vi "Teleop.vi"(10 "Match Info":T1={"Autonomous Elapsed Seconds"=0.0, "TeleOp Elapsed Seconds"=100.423, "Disabled Elapsed Seconds"=64.63, "Visited Autonomous"=FALSE, "Visited TeleOp"=TRUE, "Visited Disabled"=TRUE, "Autonomous Settings"={"Autonomous Style"=enum."Independent", "VI Refnum"=refnum}}, 11 "Call Context":T2=enum."Stop") -> ()   [LabVIEW 2015]
doc: "This VI is called for each TeleOp packet received from the DS where the robot is not disabled. It is often used to read from the joysticks and update I/O or to update setpoints for timed control loops. It should complete and return within 20 milliseconds or it may miss DS packets."
uses:
  <vilib>/Rock Robotics/WPI/DriverStation/WPI_DriverStationDerivedRobotMode.ctl
  <vilib>/Rock Robotics/WPI/DriverStation/WPI_DriverStationMatch Info.ctl
  <vilib>/Rock Robotics/WPI/Utilities/WPI_GetSetVariantRefNum.vi
  <vilib>/addons/control/pid/pid.llb/PID Output Rate Limiter (DBL).vi
  <vilib>/addons/control/pid/NI_PID_pid.lvlib
panel:
  in  "Far":dbl=0.7
  in  "Close":dbl=0.7
  in  "Target":dbl
  in  "P":dbl=1.0 format="%#_13g"
  in  "I":dbl format="%#_13g"
  in  "dT":dbl format="%#_13g"
  out "Right Chart":dbl(graph)
  out "Left Chart":dbl(graph)
  in  "dt (s)":dbl=2.0 format="%.2f"
  in  "output rate (EGU/min)":dbl=25.0 format="%.2f"
  in  "initial output":dbl format="%.2f"
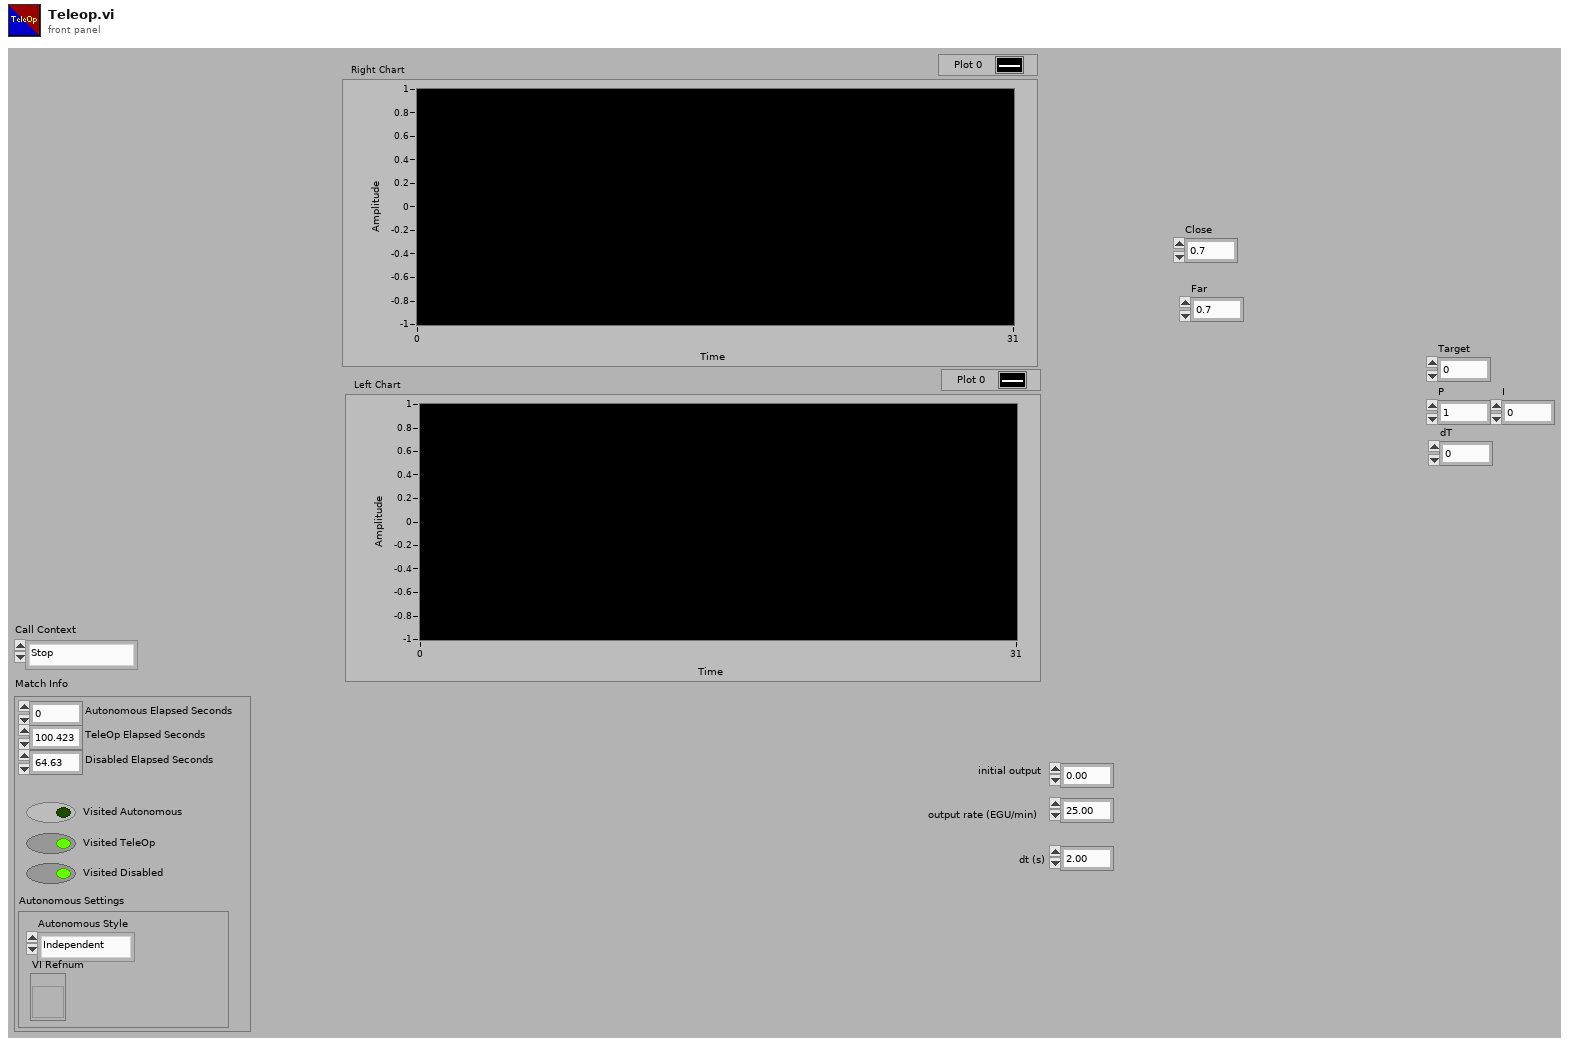
[diagram p1: front panel]
types:
  T1 = typedef "WPI_DriverStationMatch Info.ctl" = cluster{"Autonomous Elapsed Seconds":dbl, "TeleOp Elapsed Seconds":dbl, "Disabled Elapsed Seconds":dbl, "Visited Autonomous":bool, "Visited TeleOp":bool, "Visited Disabled":bool, "Autonomous Settings":cluster{"Autonomous Style":enum16{"Iterative", "Independent"}, "VI Refnum":refnum<vi>}}
  T2 = typedef "WPI_DriverStationDerivedRobotMode.ctl" = enum16{"Init", "Execute", "Stop"}
  T3 = typedef "WPI_JoystickDevRef.ctl" = cluster{"Device":T4}
  T4 = typedef "WPI_JoystickDeviceEnum.ctl" = enum16{"USB 0", "USB 1", "USB 2", "USB 3", "USB 4", "USB 5"}
  T5 = typedef "WPI_RobotDriveDevRef.ctl" = cluster{"DevStatus":errorcluster, "Motors[]":T6[], "Square Inputs":bool, "Max Output":dbl}
  T6 = typedef "WPI_MotorControlDeviceRef.ctl" = cluster{"DeviceStatus":errorcluster, "Type":T7, "PWM":cluster{"PWM Channel":T8, "DeadBand":T9}, "CAN":cluster{"Device Number":u8, "Control Mode":T10, "Semaphore":T11, "Max Vout":dbl, "TalonSRX Control Mode":T12}, "Invert":bool}
  T7 = typedef "WPI_MotorControlType.ctl" = enum16{"PWM", "CAN", "CANTalonSRX"}
  T8 = typedef "FPGA_DIOPWMChannel.ctl" = enum8{"PWM 0", "PWM 1", "PWM 2", "PWM 3", "PWM 4", "PWM 5", "PWM 6", "PWM 7", "PWM 8", "PWM 9", "PWM MXP 0", "PWM MXP 1", "PWM MXP 2", "PWM MXP 3", "PWM MXP 4", "PWM MXP 5", "PWM MXP 6", "PWM MXP 7", "PWM MXP 8", "PWM MXP 9", "Invalid"}
  T9 = typedef "WPI_PWMDeadband.ctl" = cluster{"Name":string, "maxPositivePwm":i32, "minPositivePwm":i32, "centerPwm":i32, "maxNegativePwm":i32, "minNegativePwm":i32, "angularRange":u16}
  T10 = typedef "WPI_CANJaguar_ControlMode.ctl" = enum8{"Percent VBus", "Current", "Speed", "Position", "Voltage"}
  T11 = typedef "Semaphore RefNum" = refnum<k1>
  T12 = typedef "WPI_CANTalonSRX_APIControlMode.ctl" = enum8{"Percent VBus", "Speed", "Position", "Slave", "Unchanged / Invalid", "Voltage Compensation", "Current", "Motion Profile"}
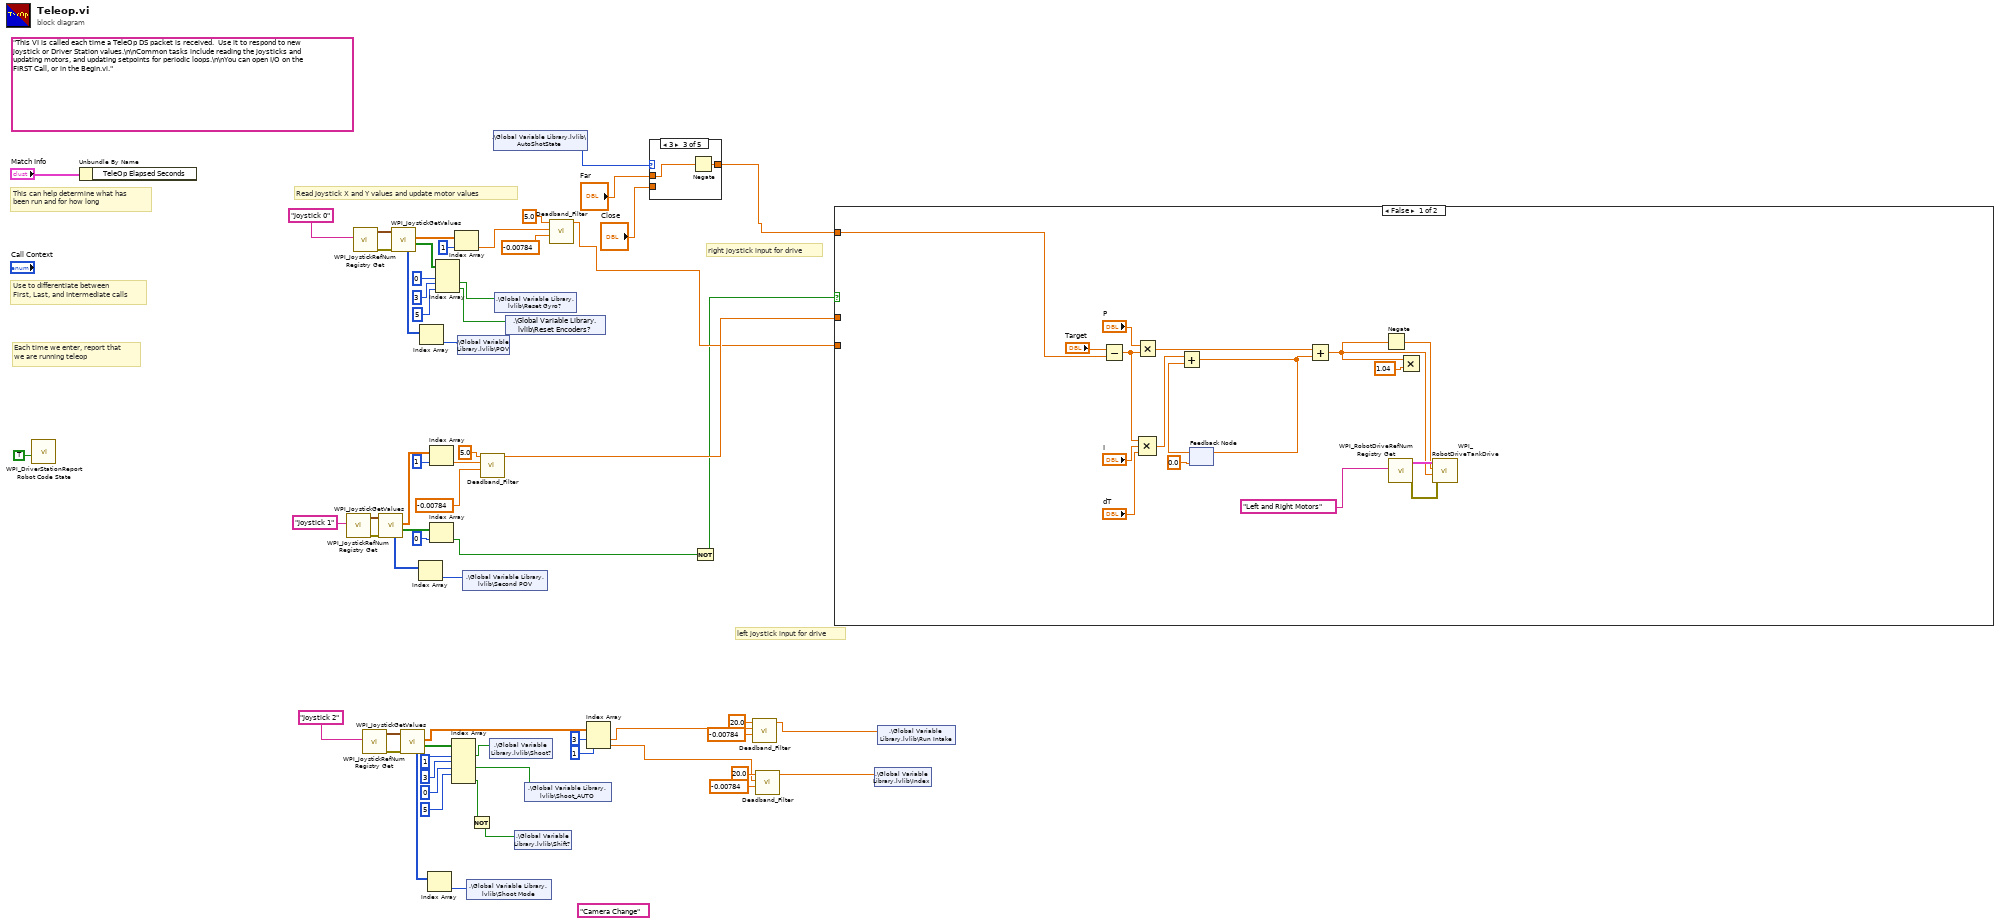
[diagram p0: block diagram]
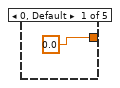
[diagram p2: hidden frame]
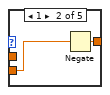
[diagram p3: hidden frame]
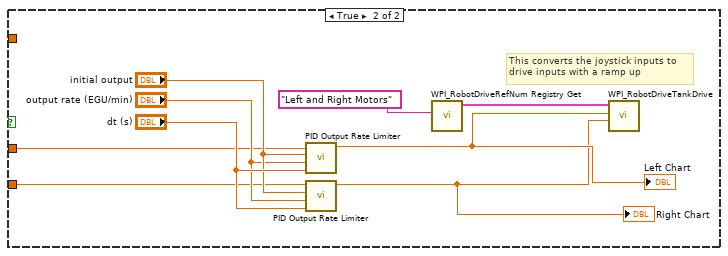
[diagram p6: hidden frame]
diagram:
  (unwired) "Camera Change" ("Name")
  (unwired) "This VI is called each time a TeleOp DS packet is received.  Use it to respond to new joystick or Driver Station values.\n\nCommon tasks include reading the joysticks and updating motors, and updating setpoints for periodic loops.\n\nYou can open I/O on the FIRST Call, or in the Begin.vi."
  # "left joystick input for drive"
  # "right joystick input for drive"
  # "Each time we enter, report that\nwe are running teleop"
  # "Use to differentiate between\nFirst, Last, and Intermediate calls"
  # "This can help determine what has\nbeen run and for how long"
  # "Read Joystick X and Y values and update motor values"
  n1 = call <vilib>:"WPI_DriverStationReport Robot Code State.vi"("TeleOp"=TRUE ("Autonomous")) -> ()  [unwired: 10 in, 1 out]
  n2 = Unbundle By Name("Match Info") -> ()  [unwired: 1 out]
  n3 = call <vilib>:"WPI_JoystickRefNum Registry Get.vi"("refnum name"="Joystick 1") -> ("error out"=w52:errorcluster, "JoystickDevRef"=w51:T3)  [unwired: 1 in, 8 out]
  n4 = call <vilib>:"WPI_JoystickRefNum Registry Get.vi"("refnum name"="Joystick 0") -> ("error out"=w58:errorcluster, "JoystickDevRef"=w57:T3)  [unwired: 1 in, 8 out]
  n5 = call <vilib>:"WPI_JoystickRefNum Registry Get.vi"("refnum name"="Joystick 2") -> ("error out"=w49:errorcluster, "JoystickDevRef"=w48:T3)  [unwired: 1 in, 8 out]
  n6 = call <vilib>:"WPI_JoystickGetValues.vi"("error in (no error)"=w52, "JoystickDevRef"=w51) -> ("Buttons"=w8:bool[], "Axes"=w50:dbl[], "POVs"=w31:i16[])  [unwired: 5 in, 2 out]
  n7 = call <vilib>:"WPI_JoystickGetValues.vi"("error in (no error)"=w58, "JoystickDevRef"=w57) -> ("Buttons"=w55:bool[], "Axes"=w56:dbl[], "POVs"=w54:i16[])  [unwired: 5 in, 2 out]
  n8 = call <vilib>:"WPI_JoystickGetValues.vi"("error in (no error)"=w49, "JoystickDevRef"=w48) -> ("Buttons"=w47:bool[], "Axes"=w27:dbl[], "POVs"=w34:i16[])  [unwired: 5 in, 2 out]
  n9 = Index Array(array=w31) -> (element=w30:i16)  [unwired: 1 in]
  n10 = Index Array(array=w54) -> (element=w53:i16)  [unwired: 1 in]
  n11 = Index Array(array=w34) -> (element=w33:i16)  [unwired: 1 in]
  n12 = Index Array(array=w50, index=1) -> (element=w40:dbl)
  n13 = Index Array(array=w8, index=0) -> (element=w6:bool)
  n14 = Index Array(array=w55, index #1=0 ("index"), index #2=3 ("index"), index #3=5 ("index")) -> (element #2=w32:bool, element #3=w14:bool)  [unwired: 1 out]
  n15 = Index Array(array=w47, index #1=1 ("index"), index #2=3 ("index"), index #3=0 ("index"), index #4=5 ("index")) -> (element #1=w46:bool, element #3=w11:bool, element #5=w10:bool)  [unwired: 1 in, 2 out]
  n16 = Index Array(array=w56, index=1) -> (element=w35:dbl)
  n17 = shared-variable ".\\Global Variable Library.lvlib\\POV"(w53) -> ()  [unwired: 1 in, 1 out]
  n18 = shared-variable ".\\Global Variable Library.lvlib\\Second POV"(w30) -> ()  [unwired: 1 in, 1 out]
  n19 = shared-variable ".\\Global Variable Library.lvlib\\Shoot Mode"(w33) -> ()  [unwired: 1 in, 1 out]
  n20 = Not(x=w10) -> (.not. x?=w9:bool)
  n21 = call "Deadband_Filter.vi"("Deadband_Center"=-0.00784, "Input"=w40, "Deadband_Size(%)"=5.0) -> ("Deadbanded_Output"=w13:dbl)  [unwired: 8 in]
  n22 = shared-variable ".\\Global Variable Library.lvlib\\Shoot?"(w46) -> ()  [unwired: 1 in, 1 out]
  n23 = shared-variable ".\\Global Variable Library.lvlib\\AutoShotState"() -> (w3:u32)  [unwired: 1 in, 1 out]
  n24 = shared-variable ".\\Global Variable Library.lvlib\\Reset Gyro?"(w32) -> ()  [unwired: 1 in, 1 out]
  n25 = shared-variable ".\\Global Variable Library.lvlib\\Reset Encoders?"(w14) -> ()  [unwired: 1 in, 1 out]
  n26 = shared-variable ".\\Global Variable Library.lvlib\\Shift?"(w9) -> ()  [unwired: 1 in, 1 out]
  n27 = shared-variable ".\\Global Variable Library.lvlib\\Shoot_AUTO"(w11) -> ()  [unwired: 1 in, 1 out]
  n28 = call "Deadband_Filter.vi"("Deadband_Center"=-0.00784, "Input"=w35, "Deadband_Size(%)"=5.0) -> ("Deadbanded_Output"=w12:dbl)  [unwired: 8 in]
  n29 = Index Array(array=w27, index #1=3 ("index"), index #2=1 ("index")) -> (element #1=w20:dbl, element #2=w17:dbl)
  n30 = case shown="3" w3 {
    tunnel: [0.0 w66 w68 w69 w70] -> w4
    tunnel: "Far" -> [_ _ w67 _ w70]
    tunnel: "Close" -> [_ w65 _ w69 _]
    frame 0, Default {
    }
    frame 1 {
      n31 = Negate(x=w65) -> (-x=w66:dbl)
    }
    frame 3 {
      n32 = Negate(x=w67) -> (-x=w68:dbl)
    }
    frame 4 {
    }
    frame 6 {
    }
  }
  n33 = Not(x=w6) -> (.not. x?=w5:bool)
  n34 = call "Deadband_Filter.vi"("Deadband_Center"=-0.00784, "Input"=w20, "Deadband_Size(%)"=20.0) -> ("Deadbanded_Output"=w21:dbl)  [unwired: 8 in]
  n35 = call "Deadband_Filter.vi"("Deadband_Center"=-0.00784, "Input"=w17, "Deadband_Size(%)"=20.0) -> ("Deadbanded_Output"=w16:dbl)  [unwired: 8 in]
  n36 = case shown="False" w5 {
    tunnel: w13 -> [_ w91]
    tunnel: w12 -> [_ w90]
    tunnel: w4 -> [w73 _]
    frame False {
      n37 = Subtract(x="Target", y=w73) -> (x-y=w81:dbl)
      n38 = Multiply(x="P", y=w81) -> (x*y=w84:dbl)
      n39 = Compound Arithmetic op=MULTIPLY(w81, "I", "dT") -> (w76:dbl)
      n40 = feedback #1(0.0) -> (w77:dbl)
      n41 = Add(x=w76, y=w77) -> (x+y=w78:dbl)
      n42 = feedback-in #1(w78) -> ()
      n43 = Add(x=w84, y=w78) -> (x+y=w72:dbl)
      n44 = Negate(x=w72) -> (-x=w71:dbl)
      n45 = call <vilib>:"WPI_RobotDriveRefNum Registry Get.vi"("refnum name"="Left and Right Motors") -> ("error out"=w86:errorcluster, "RobotDriveDevRef"=w85:T5)  [unwired: 9 in]
      n46 = Multiply(x=w72, y=1.04) -> ()  [unwired: 1 out]
      n47 = call <vilib>:"WPI_RobotDriveTankDrive.vi"("error in (no error)"=w86, "Right axis value"=w72, "Left axis value"=w71, "RobotDriveDevRef"=w85) -> ()  [unwired: 5 in, 3 out]
    }
    frame True {
      # "This converts the joystick inputs to\ndrive inputs with a ramp up"
      n48 = call-poly <vilib>:"PID Output Rate Limiter.vi"("dt (s)"="dt (s)", "output rate (EGU/min)"="output rate (EGU/min)", "initial output"="initial output", "input (controller output)"=w91) -> ("output"=w89:dbl)  [unwired: 4 in, 1 out]
      "Left Chart" <- w89
      n49 = call-poly <vilib>:"PID Output Rate Limiter.vi"("dt (s)"="dt (s)", "output rate (EGU/min)"="output rate (EGU/min)", "initial output"="initial output", "input (controller output)"=w90) -> ("output"=w88:dbl)  [unwired: 4 in, 1 out]
      "Right Chart" <- w88
      n50 = call <vilib>:"WPI_RobotDriveRefNum Registry Get.vi"("refnum name"="Left and Right Motors") -> ("RobotDriveDevRef"=w95:T5)  [unwired: 9 in, 1 out]
      n51 = call <vilib>:"WPI_RobotDriveTankDrive.vi"("Right axis value"=w88, "Left axis value"=w89, "RobotDriveDevRef"=w95) -> ()  [unwired: 6 in, 3 out]
    }
  }
  n52 = shared-variable ".\\Global Variable Library.lvlib\\Index"(w16) -> ()  [unwired: 1 in, 1 out]
  n53 = shared-variable ".\\Global Variable Library.lvlib\\Run Intake"(w21) -> ()  [unwired: 1 in, 1 out]
